vi "Create Display Resources.vi"(0 "common resources":T5) -> (4 "display channel resources":T4)   [LabVIEW 2020, in "GettingStarted_Common_148X_FPGA.lvlib"]
uses:
  GettingStarted_Common_148X_FPGA.lvlib
  Types/Common Resources.ctl
  <instrlib>/_niInstr/Memory/v1/FPGA/DRAM/niInstr Memory DRAM v1 FPGA.lvclass
  <instrlib>/FlexRIO/CSI-2/v2/FPGA/Types/Sync Pulse Resources.ctl
  Types/Serial Channel Resources.ctl
  Types/Single Serial Channel Resources.ctl
  <instrlib>/FlexRIO/CSI-2/v2/FPGA/DRAM Manager/Private/DRAM Manager.ctl
  <instrlib>/FlexRIO/CSI-2/v2/FPGA/DRAM Manager/Private/Common/DRAM Manager Registers.ctl
  <instrlib>/FlexRIO/CSI-2/v2/FPGA/DRAM Manager/Private/Common/Handshake Registers.ctl
  <instrlib>/FlexRIO/CSI-2/v2/FPGA/DRAM Manager/Private/Common/DRAM Manager FIFOs.ctl
  <instrlib>/FlexRIO/CSI-2/v2/FPGA/DRAM Manager/Private/Common/Write Data FIFO Ref.ctl
  <instrlib>/FlexRIO/CSI-2/v2/FPGA/DRAM Manager/Private/Common/Read Request Metadata FIFO Ref.ctl
  <instrlib>/FlexRIO/CSI-2/v2/FPGA/DRAM Manager/Private/Common/Read Data FIFO Ref.ctl
  Types/Display Channel Resources.ctl
  <instrlib>/FlexRIO/CSI-2/v2/FPGA/NI CSI-2 API FPGA v2.lvlib
  <instrlib>/FlexRIO/CSI-2/v2/FPGA/DRAM Manager/DRAM Manager v2.lvlib
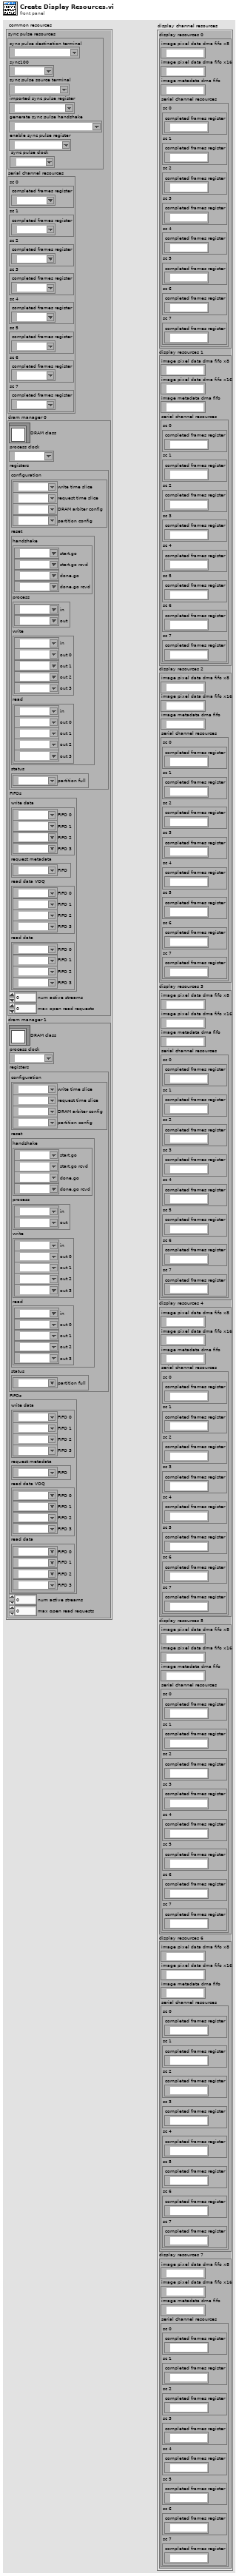
[diagram p1: front panel]
types:
  T1 = typedef "GettingStarted_Common_148X_FPGA.lvlib/Display Channel Resources.ctl" = cluster{"image pixel data dma fifo x8":refnum<k21>, "image pixel data dma fifo x16":refnum<k21>, "image metadata dma fifo":refnum<k21>, "serial channel resources":T2}
  T2 = typedef "GettingStarted_Common_148X_FPGA.lvlib/Serial Channel Resources.ctl" = cluster{"sc 0":T3, "sc 1":T3, "sc 2":T3, "sc 3":T3, "sc 4":T3, "sc 5":T3, "sc 6":T3, "sc 7":T3}
  T3 = typedef "GettingStarted_Common_148X_FPGA.lvlib/Single Serial Channel Resources.ctl" = cluster{"completed frames register":refnum<k21>}
  T4 = cluster{"display resources 0":T1, "display resources 1":T1, "display resources 2":T1, "display resources 3":T1, "display resources 4":T1, "display resources 5":T1, "display resources 6":T1, "display resources 7":T1}
  T5 = typedef "GettingStarted_Common_148X_FPGA.lvlib/Common Resources.ctl" = cluster{"sync pulse resources":T6, "serial channel resources":T2, "dram manager 0":T7, "dram manager 1":T7}
  T6 = typedef "NI CSI-2 API FPGA v2.lvlib/Sync Pulse Resources.ctl" = cluster{"sync pulse destination terminal":refnum<k21>, "sync100":refnum<k21>, "sync pulse source terminal":refnum<k21>, "imported sync pulse register":refnum<k21>, "generate sync pulse handshake":refnum<k21>, "enable sync pulse register":refnum<k21>, "sync pulse clock":refnum<k21>}
  T7 = typedef "DRAM Manager v2.lvlib/DRAM Manager.ctl" = cluster{"DRAM class":refnum<class "niInstr Memory DRAM v1 FPGA.lvclass">, "process clock":refnum<k21>, "registers":T8, "FIFOs":T10, "num active streams":fxp<+,3,3>, "max open read requests":u16}
  T8 = typedef "DRAM Manager v2.lvlib/DRAM Manager Registers.ctl" = cluster{"configuration":cluster{"write time slice":refnum<k21>, "request time slice":refnum<k21>, "DRAM arbiter config":refnum<k21>, "partition config":refnum<k21>}, "reset":cluster{"handshake":T9, "process":cluster{"in":refnum<k21>, "out":refnum<k21>}, "write":cluster{"in":refnum<k21>, "out 0":refnum<k21>, "out 1":refnum<k21>, "out 2":refnum<k21>, "out 3":refnum<k21>}, "read":cluster{"in":refnum<k21>, "out 0":refnum<k21>, "out 1":refnum<k21>, "out 2":refnum<k21>, "out 3":refnum<k21>}}, "status":cluster{"partition full":refnum<k21>}}
  T9 = typedef "DRAM Manager v2.lvlib/Handshake Registers.ctl" = cluster{"start.go":refnum<k21>, "start.go rcvd":refnum<k21>, "done.go":refnum<k21>, "done.go rcvd":refnum<k21>}
  T10 = typedef "DRAM Manager v2.lvlib/DRAM Manager FIFOs.ctl" = cluster{"write data":cluster{"FIFO 0":T11, "FIFO 1":T11, "FIFO 2":T11, "FIFO 3":T11}, "request metadata":cluster{"FIFO":T12}, "read data VOQ":cluster{"FIFO 0":T13, "FIFO 1":T13, "FIFO 2":T13, "FIFO 3":T13}, "read data":cluster{"FIFO 0":T13, "FIFO 1":T13, "FIFO 2":T13, "FIFO 3":T13}}
  T11 = typedef "DRAM Manager v2.lvlib/Write Data FIFO Ref.ctl" = refnum<k21>
  T12 = typedef "DRAM Manager v2.lvlib/Read Request Metadata FIFO Ref.ctl" = refnum<k21>
  T13 = typedef "DRAM Manager v2.lvlib/Read Data FIFO Ref.ctl" = refnum<k21>
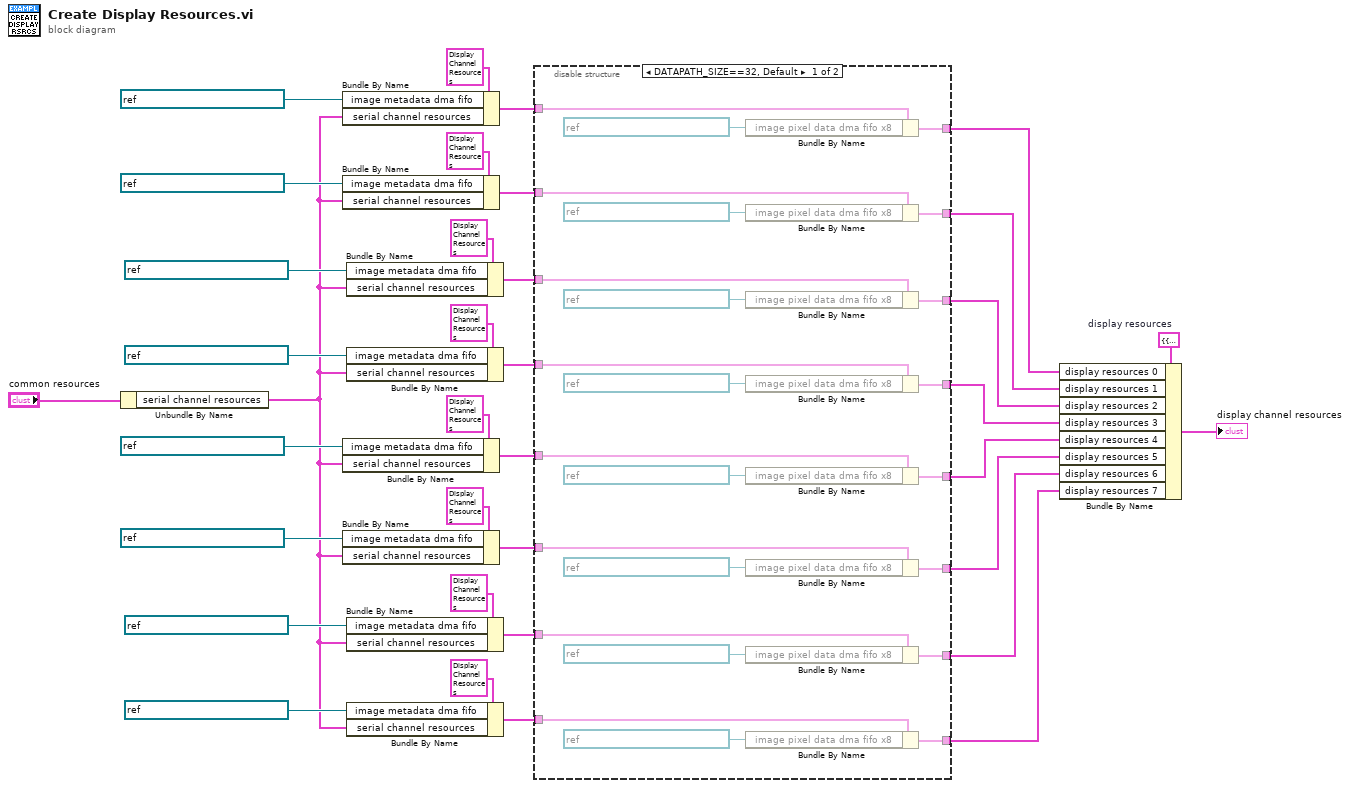
[diagram p0: block diagram]
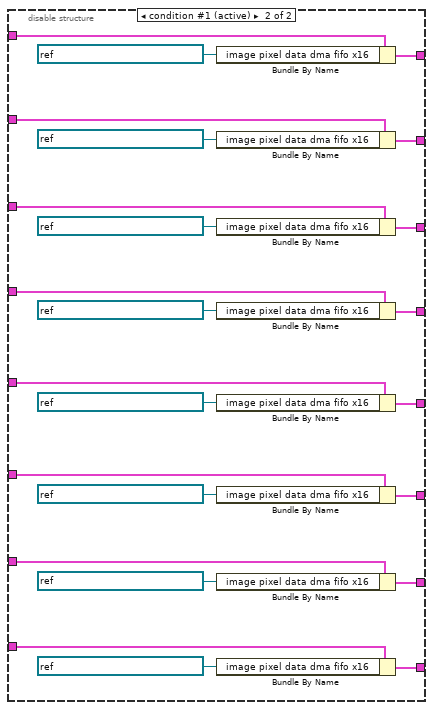
[diagram p2: hidden frame]
diagram:
  w27 = T4 {"display resources 0"={"image pixel data dma fifo x8"="", "image pixel data dma fifo x16"="", "image metadata dma fifo"="", "serial channel resources"={"sc 0"={"completed frames register"=""}, "sc 1"={"completed frames register"=""}, "sc 2"={"completed frames register"=""}, "sc 3"={"completed frames register"=""}, "sc 4"={"completed frames register"=""}, "sc 5"={"completed frames register"=""}, "sc 6"={"completed frames register"=""}, "sc 7"={"completed frames register"=""}}}, "display resources 1"={"image pixel data dma fifo x8"="", "image pixel data dma fifo x16"="", "image metadata dma fifo"="", "serial channel resources"={"sc 0"={"completed frames register"=""}, "sc 1"={"completed frames register"=""}, "sc 2"={"completed frames register"=""}, "sc 3"={"completed frames register"=""}, "sc 4"={"completed frames register"=""}, "sc 5"={"completed frames register"=""}, "sc 6"={"completed frames register"=""}, "sc 7"={"completed frames register"=""}}}, "display resources 2"={"image pixel data dma fifo x8"="", "image pixel data dma fifo x16"="", "image metadata dma fifo"="", "serial channel resources"={"sc 0"={"completed frames register"=""}, "sc 1"={"completed frames register"=""}, "sc 2"={"completed frames register"=""}, "sc 3"={"completed frames register"=""}, "sc 4"={"completed frames register"=""}, "sc 5"={"completed frames register"=""}, "sc 6"={"completed frames register"=""}, "sc 7"={"completed frames register"=""}}}, "display resources 3"={"image pixel data dma fifo x8"="", "image pixel data dma fifo x16"="", "image metadata dma fifo"="", "serial channel resources"={"sc 0"={"completed frames register"=""}, "sc 1"={"completed frames register"=""}, "sc 2"={"completed frames register"=""}, "sc 3"={"completed frames register"=""}, "sc 4"={"completed frames register"=""}, "sc 5"={"completed frames register"=""}, "sc 6"={"completed frames register"=""}, "sc 7"={"completed frames register"=""}}}, "display resources 4"={"image pixel data dma fifo x8"="", "image pixel data dma fifo x16"="", "image metadata dma fifo"="", "serial channel resources"={"sc 0"={"completed frames register"=""}, "sc 1"={"completed frames register"=""}, "sc 2"={"completed frames register"=""}, "sc 3"={"completed frames register"=""}, "sc 4"={"completed frames register"=""}, "sc 5"={"completed frames register"=""}, "sc 6"={"completed frames register"=""}, "sc 7"={"completed frames register"=""}}}, "display resources 5"={"image pixel data dma fifo x8"="", "image pixel data dma fifo x16"="", "image metadata dma fifo"="", "serial channel resources"={"sc 0"={"completed frames register"=""}, "sc 1"={"completed frames register"=""}, "sc 2"={"completed frames register"=""}, "sc 3"={"completed frames register"=""}, "sc 4"={"completed frames register"=""}, "sc 5"={"completed frames register"=""}, "sc 6"={"completed frames register"=""}, "sc 7"={"completed frames register"=""}}}, "display resources 6"={"image pixel data dma fifo x8"="", "image pixel data dma fifo x16"="", "image metadata dma fifo"="", "serial channel resources"={"sc 0"={"completed frames register"=""}, "sc 1"={"completed frames register"=""}, "sc 2"={"completed frames register"=""}, "sc 3"={"completed frames register"=""}, "sc 4"={"completed frames register"=""}, "sc 5"={"completed frames register"=""}, "sc 6"={"completed frames register"=""}, "sc 7"={"completed frames register"=""}}}, "display resources 7"={"image pixel data dma fifo x8"="", "image pixel data dma fifo x16"="", "image metadata dma fifo"="", "serial channel resources"={"sc 0"={"completed frames register"=""}, "sc 1"={"completed frames register"=""}, "sc 2"={"completed frames register"=""}, "sc 3"={"completed frames register"=""}, "sc 4"={"completed frames register"=""}, "sc 5"={"completed frames register"=""}, "sc 6"={"completed frames register"=""}, "sc 7"={"completed frames register"=""}}}}  # display resources
  n1 = Unbundle By Name("common resources") -> ("serial channel resources"=w17:T2)
  n2 = Bundle By Name(cluster=T1 {"image pixel data dma fifo x8"="", "image pixel data dma fifo x16"="", "image metadata dma fifo"="", "serial channel resources"={"sc 0"={"completed frames register"=""}, "sc 1"={"completed frames register"=""}, "sc 2"={"completed frames register"=""}, "sc 3"={"completed frames register"=""}, "sc 4"={"completed frames register"=""}, "sc 5"={"completed frames register"=""}, "sc 6"={"completed frames register"=""}, "sc 7"={"completed frames register"=""}}} ("display resources"), "image metadata dma fifo"=refnum<k21> "Display 0 Image Metadata", "serial channel resources"=w17) -> (w14:T1)
  n3 = Bundle By Name(cluster=T1 {"image pixel data dma fifo x8"="", "image pixel data dma fifo x16"="", "image metadata dma fifo"="", "serial channel resources"={"sc 0"={"completed frames register"=""}, "sc 1"={"completed frames register"=""}, "sc 2"={"completed frames register"=""}, "sc 3"={"completed frames register"=""}, "sc 4"={"completed frames register"=""}, "sc 5"={"completed frames register"=""}, "sc 6"={"completed frames register"=""}, "sc 7"={"completed frames register"=""}}} ("display resources"), "image metadata dma fifo"=refnum<k21> "Display 1 Image Metadata", "serial channel resources"=w17) -> (w12:T1)
  n4 = Bundle By Name(cluster=T1 {"image pixel data dma fifo x8"="", "image pixel data dma fifo x16"="", "image metadata dma fifo"="", "serial channel resources"={"sc 0"={"completed frames register"=""}, "sc 1"={"completed frames register"=""}, "sc 2"={"completed frames register"=""}, "sc 3"={"completed frames register"=""}, "sc 4"={"completed frames register"=""}, "sc 5"={"completed frames register"=""}, "sc 6"={"completed frames register"=""}, "sc 7"={"completed frames register"=""}}} ("display resources"), "image metadata dma fifo"=refnum<k21> "Display 4 Image Metadata", "serial channel resources"=w17) -> (w8:T1)
  n5 = Bundle By Name(cluster=T1 {"image pixel data dma fifo x8"="", "image pixel data dma fifo x16"="", "image metadata dma fifo"="", "serial channel resources"={"sc 0"={"completed frames register"=""}, "sc 1"={"completed frames register"=""}, "sc 2"={"completed frames register"=""}, "sc 3"={"completed frames register"=""}, "sc 4"={"completed frames register"=""}, "sc 5"={"completed frames register"=""}, "sc 6"={"completed frames register"=""}, "sc 7"={"completed frames register"=""}}} ("display resources"), "image metadata dma fifo"=refnum<k21> "Display 5 Image Metadata", "serial channel resources"=w17) -> (w6:T1)
  n6 = Bundle By Name(cluster=T1 {"image pixel data dma fifo x8"="", "image pixel data dma fifo x16"="", "image metadata dma fifo"="", "serial channel resources"={"sc 0"={"completed frames register"=""}, "sc 1"={"completed frames register"=""}, "sc 2"={"completed frames register"=""}, "sc 3"={"completed frames register"=""}, "sc 4"={"completed frames register"=""}, "sc 5"={"completed frames register"=""}, "sc 6"={"completed frames register"=""}, "sc 7"={"completed frames register"=""}}} ("display resources"), "image metadata dma fifo"=refnum<k21> "Display 2 Image Metadata", "serial channel resources"=w17) -> (w10:T1)
  n7 = Bundle By Name(cluster=T1 {"image pixel data dma fifo x8"="", "image pixel data dma fifo x16"="", "image metadata dma fifo"="", "serial channel resources"={"sc 0"={"completed frames register"=""}, "sc 1"={"completed frames register"=""}, "sc 2"={"completed frames register"=""}, "sc 3"={"completed frames register"=""}, "sc 4"={"completed frames register"=""}, "sc 5"={"completed frames register"=""}, "sc 6"={"completed frames register"=""}, "sc 7"={"completed frames register"=""}}} ("display resources"), "image metadata dma fifo"=refnum<k21> "Display 3 Image Metadata", "serial channel resources"=w17) -> (w16:T1)
  n8 = Bundle By Name(cluster=T1 {"image pixel data dma fifo x8"="", "image pixel data dma fifo x16"="", "image metadata dma fifo"="", "serial channel resources"={"sc 0"={"completed frames register"=""}, "sc 1"={"completed frames register"=""}, "sc 2"={"completed frames register"=""}, "sc 3"={"completed frames register"=""}, "sc 4"={"completed frames register"=""}, "sc 5"={"completed frames register"=""}, "sc 6"={"completed frames register"=""}, "sc 7"={"completed frames register"=""}}} ("display resources"), "image metadata dma fifo"=refnum<k21> "Display 6 Image Metadata", "serial channel resources"=w17) -> (w4:T1)
  n9 = Bundle By Name(cluster=T1 {"image pixel data dma fifo x8"="", "image pixel data dma fifo x16"="", "image metadata dma fifo"="", "serial channel resources"={"sc 0"={"completed frames register"=""}, "sc 1"={"completed frames register"=""}, "sc 2"={"completed frames register"=""}, "sc 3"={"completed frames register"=""}, "sc 4"={"completed frames register"=""}, "sc 5"={"completed frames register"=""}, "sc 6"={"completed frames register"=""}, "sc 7"={"completed frames register"=""}}} ("display resources"), "image metadata dma fifo"=refnum<k21> "Display 7 Image Metadata", "serial channel resources"=w17) -> (w2:T1)
  n10 = disable-structure shown="DATAPATH_SIZE==32, Default" {
    disable-tunnel: w16 -> [w59 w83]
    disable-tunnel: [w58 w82] -> w15
    disable-tunnel: w14 -> [w56 w80]
    disable-tunnel: [w55 w79] -> w13
    disable-tunnel: w12 -> [w53 w77]
    disable-tunnel: [w52 w76] -> w11
    disable-tunnel: w10 -> [w50 w74]
    disable-tunnel: [w49 w73] -> w9
    disable-tunnel: w8 -> [w47 w71]
    disable-tunnel: [w46 w70] -> w7
    disable-tunnel: w6 -> [w44 w68]
    disable-tunnel: [w43 w67] -> w5
    disable-tunnel: w4 -> [w41 w65]
    disable-tunnel: [w40 w64] -> w3
    disable-tunnel: w2 -> [w39 w63]
    disable-tunnel: [w38 w62] -> w1
    frame condition #0 {
      n11 = Bundle By Name(cluster=w56, "image pixel data dma fifo x8"=refnum<k21> "Display 0 Image Pixel Data" ("image pixel data dma fifo")) -> (w55:T1)
      n12 = Bundle By Name(cluster=w53, "image pixel data dma fifo x8"=refnum<k21> "Display 1 Image Pixel Data" ("image pixel data dma fifo")) -> (w52:T1)
      n13 = Bundle By Name(cluster=w50, "image pixel data dma fifo x8"=refnum<k21> "Display 2 Image Pixel Data" ("image pixel data dma fifo")) -> (w49:T1)
      n14 = Bundle By Name(cluster=w59, "image pixel data dma fifo x8"=refnum<k21> "Display 3 Image Pixel Data" ("image pixel data dma fifo")) -> (w58:T1)
      n15 = Bundle By Name(cluster=w47, "image pixel data dma fifo x8"=refnum<k21> "Display 4 Image Pixel Data" ("image pixel data dma fifo")) -> (w46:T1)
      n16 = Bundle By Name(cluster=w44, "image pixel data dma fifo x8"=refnum<k21> "Display 5 Image Pixel Data" ("image pixel data dma fifo")) -> (w43:T1)
      n17 = Bundle By Name(cluster=w41, "image pixel data dma fifo x8"=refnum<k21> "Display 6 Image Pixel Data" ("image pixel data dma fifo")) -> (w40:T1)
      n18 = Bundle By Name(cluster=w39, "image pixel data dma fifo x8"=refnum<k21> "Display 7 Image Pixel Data" ("image pixel data dma fifo")) -> (w38:T1)
    }
    frame condition #1 (active) {
      n19 = Bundle By Name(cluster=w80, "image pixel data dma fifo x16"=refnum<k21> "Display 0 Image Pixel Data" ("image pixel data dma fifo")) -> (w79:T1)
      n20 = Bundle By Name(cluster=w77, "image pixel data dma fifo x16"=refnum<k21> "Display 1 Image Pixel Data" ("image pixel data dma fifo")) -> (w76:T1)
      n21 = Bundle By Name(cluster=w74, "image pixel data dma fifo x16"=refnum<k21> "Display 2 Image Pixel Data" ("image pixel data dma fifo")) -> (w73:T1)
      n22 = Bundle By Name(cluster=w83, "image pixel data dma fifo x16"=refnum<k21> "Display 3 Image Pixel Data" ("image pixel data dma fifo")) -> (w82:T1)
      n23 = Bundle By Name(cluster=w71, "image pixel data dma fifo x16"=refnum<k21> "Display 4 Image Pixel Data" ("image pixel data dma fifo")) -> (w70:T1)
      n24 = Bundle By Name(cluster=w68, "image pixel data dma fifo x16"=refnum<k21> "Display 5 Image Pixel Data" ("image pixel data dma fifo")) -> (w67:T1)
      n25 = Bundle By Name(cluster=w65, "image pixel data dma fifo x16"=refnum<k21> "Display 6 Image Pixel Data" ("image pixel data dma fifo")) -> (w64:T1)
      n26 = Bundle By Name(cluster=w63, "image pixel data dma fifo x16"=refnum<k21> "Display 7 Image Pixel Data" ("image pixel data dma fifo")) -> (w62:T1)
    }
  }
  n27 = Bundle By Name(cluster=w27, "display resources 0"=w13, "display resources 1"=w11, "display resources 2"=w9, "display resources 3"=w15, "display resources 4"=w7, "display resources 5"=w5, "display resources 6"=w3, "display resources 7"=w1) -> (→"display channel resources":T4)
